vi "Get All Channel Gains.vi"(8 "error in (no error)":errorcluster, 11 "Channel Params []":T1[](array[typedef]) {"channel" min=1 max=8 step=1}) -> (0 "error out":errorcluster, 3 "Gains []":dbl[](array[numeric]))   [LabVIEW 2019, in "KH7008.lvlib"]
uses:
  KH7008.lvlib
  typedefs/channelProperties--Cluster.ctl
  typedefs/channel--numeric.ctl
  typedefs/gain--enum.ctl
  typedefs/Input--Enum.ctl
  typedefs/shunt--enum.ctl
  typedefs/couple--Enum.ctl
  typedefs/Filter--Enum.ctl
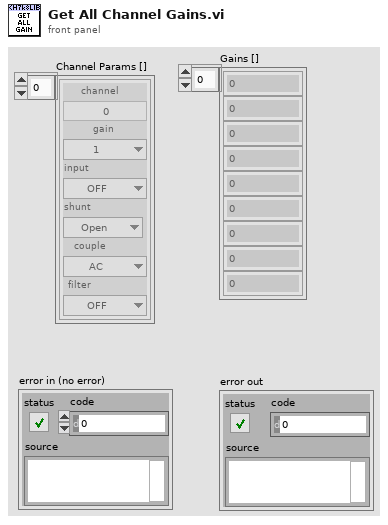
[diagram p1: front panel]
types:
  T1 = typedef "KH7008.lvlib/channelProperties--Cluster.ctl" = cluster{"channel":T2, "gain":T3, "input":T4, "shunt":T5, "couple":T6, "filter":T7}
  T2 = typedef "KH7008.lvlib/channel--numeric.ctl" = u16
  T3 = typedef "KH7008.lvlib/gain--enum.ctl" = enum16{"1", "10", "100", "1000"}
  T4 = typedef "KH7008.lvlib/input--enum.ctl" = enum16{"OFF", "SE+", "SE-", "DIFF"}
  T5 = typedef "KH7008.lvlib/shunt--enum.ctl" = enum16{"Open", "50", "500", "5k", "50k", "10M"}
  T6 = typedef "KH7008.lvlib/couple--enum.ctl" = enum16{"AC", "DC"}
  T7 = typedef "KH7008.lvlib/filter--enum.ctl" = enum16{"OFF", "ON"}
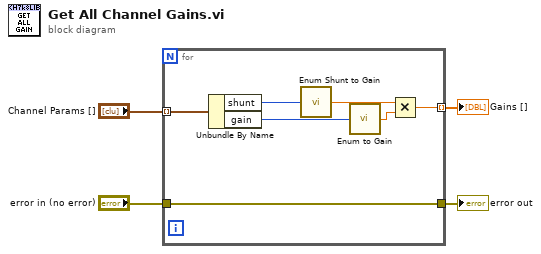
[diagram p0: block diagram]
diagram:
  n1 = for {
    tunnel: "Channel Params []" -> [w8] mode=indexing
    tunnel: [w11] -> w1 mode=indexing
    tunnel: "error in (no error)" -> [w5]
    tunnel: [w5] -> w3
    n2 = Unbundle By Name(w8) -> ("shunt"=w7:T5, "gain"=w6:T3)
    n3 = call "Enum Shunt to Gain.vi"("Shunt Resistor"=w7) -> ("Gain (V/A)"=w10:dbl)
    n4 = call "Enum to Gain.vi"("Gain"=w6) -> ("Gain (x)"=w9:dbl)
    n5 = Multiply(x=w10, y=w9) -> (x*y=w11:dbl)
  }
  "error out" <- w3
  "Gains []" <- w1
